vi "FPGA_AIReadAverageBits.vi"(8 "error in (no error)":errorcluster, 10 "Channel":T1=enum."AI 1", 11 "AI Reference in":T2) -> (0 "error out":errorcluster, 2 "AverageBits":u8, 3 "AI Reference out":T2)   [LabVIEW 2017]
uses:
  <vilib>/Rock Robotics/SystemInterfaces/AI/FPGA_AIDevRef.ctl
  <vilib>/Rock Robotics/SystemInterfaces/AI/FPGA_AIChannel.ctl
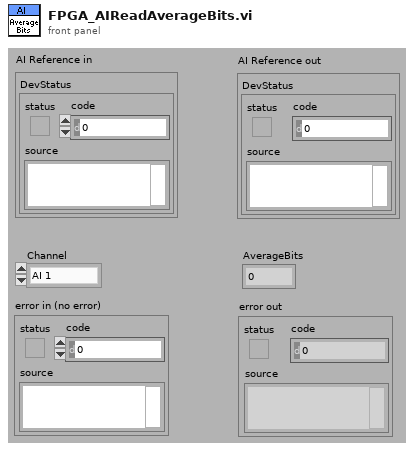
[diagram p1: front panel]
types:
  T1 = typedef "FPGA_AIChannel.ctl" = enum8{"AI 0", "AI 1", "AI 2", "AI 3", "AI MXP 0", "AI MXP 1", "AI MXP 2", "AI MXP 3", "Invalid"}
  T2 = typedef "FPGA_AIDevRef.ctl" = cluster{"DevStatus":errorcluster}
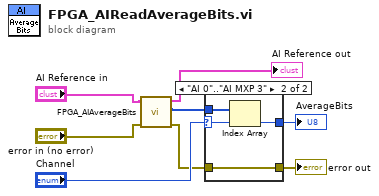
[diagram p0: block diagram]
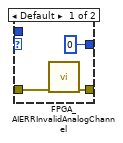
[diagram p2: hidden frame]
diagram:
  n1 = call <vilib>:"FPGA_AIAverageBits.vi"("error in (no error)"="error in (no error)", "AI Reference in"="AI Reference in") -> ("error out"=w1:errorcluster, "AverageBits out"=w4:u8[], "AI Reference out"=→"AI Reference out":T2)  [unwired: 2 in, 5 out]
  n2 = case shown="\"AI 0\"..\"AI MXP 3\"" "Channel" {
    selector: "Channel" -> [_ w15]
    tunnel: [u8 0 ("AverageBits") w14] -> w7
    tunnel: w4 -> [_ w13]
    tunnel: [w10 w12] -> w2
    tunnel: w1 -> [w9 w12]
    frame Default {
      n3 = call <vilib>:"FPGA_AIERRInvalidAnalogChannel.vi"("error in (no error)"=w9) -> ("error out"=w10:errorcluster)  [unwired: 10 in]
    }
    frame "AI 0".."AI MXP 3" {
      n4 = Index Array(array=w13, index=w15) -> (element=w14:u8)
    }
  }
  "AverageBits" <- w7
  "error out" <- w2
